vi "Create Iterator.vi"(8 "error in (no error)":errorcluster caption="错误输入（无错误）", 11 "聚集（抽象类） 输入":refnum<class "聚集（抽象类）.lvclass"> caption="DNL_LabVIEW Object in") -> (0 "error out":errorcluster caption="错误输出", 2 "迭代器.lvlib:迭代器(抽象类).lvclass":refnum<class "迭代器(抽象类).lvclass">, 3 "聚集（抽象类） 输出":refnum<class "聚集（抽象类）.lvclass"> caption="DNL_LabVIEW Object out")   [LabVIEW 2011, in "迭代器.lvlib" / "聚集（抽象类）.lvclass"]
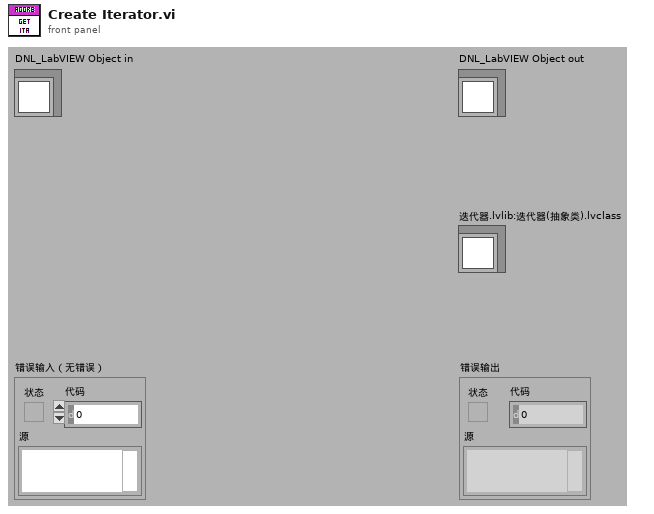
[diagram p1: front panel]
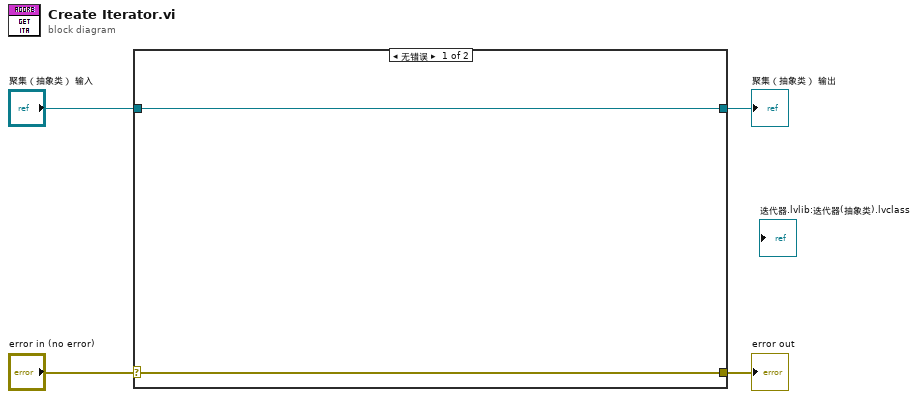
[diagram p0: block diagram]
diagram:
  n1 = case shown="无错误" "error in (no error)" {
    selector: "error in (no error)" -> [w5 w8]
    tunnel: [w5 w8] -> w3
    tunnel: [w6 w7] -> w1
    tunnel: "聚集（抽象类） 输入" -> [w6 w7]
    frame No Error {
    }
    frame Error {
    }
  }
  "error out" <- w3
  "聚集（抽象类） 输出" <- w1
